vi "Stop Core.vi"(10 "final error code":i32, 11 "ConnectionFactoryHandler in":refnum<class "ConnectionFactoryHandler.lvclass">) -> (3 "ConnectionFactoryHandler out":refnum<class "ConnectionFactoryHandler.lvclass">)   [LabVIEW 2019, in "ConnectionFactorySession.lvlib" / "ConnectionFactoryHandler.lvclass"]
doc: "(<B>Filename</B>: Actor Framework.lvlib:Actor.lvclass:Stop Core.vi)\n\nDefines what the actor does before it stops. Use the <B>final error code</B> input to determine whether the actor shut down in response to an error.\n\nBy default, this method does nothing. A descendant class may override it to define behavior, such as shutting down any processes the actor initiated in its override of the Actor Core method."
uses:
  <vilib>/gpm_packages/@cs/Network-interface/Source/Connection Factory Session/ConnectionFactoryHandler/ConnectionFactoryHandler.lvclass
  <vilib>/gpm_packages/@cs/Network-interface/Source/Connection Factory Session/ConnectionFactoryHandler/ConnectionFactoryHandler.lvclass/ConnectionFactoryHandler.ctl
  <vilib>/gpm_packages/@cs/Network-interface/Source/IConnectionFactory/IConnectionFactory.lvclass
  <vilib>/gpm_packages/@cs/Network-interface/Source/Connection Factory Session/INewConnectionCallback/INewConnectionCallback.lvclass
  <vilib>/gpm_packages/@cs/Network-interface/Source/Logged Actor/LoggedActor.lvclass
  <vilib>/gpm_packages/@cs/Network-interface/Source/Connection Reference/Connection Reference/Connection Reference.lvclass
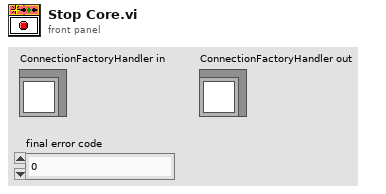
[diagram p1: front panel]
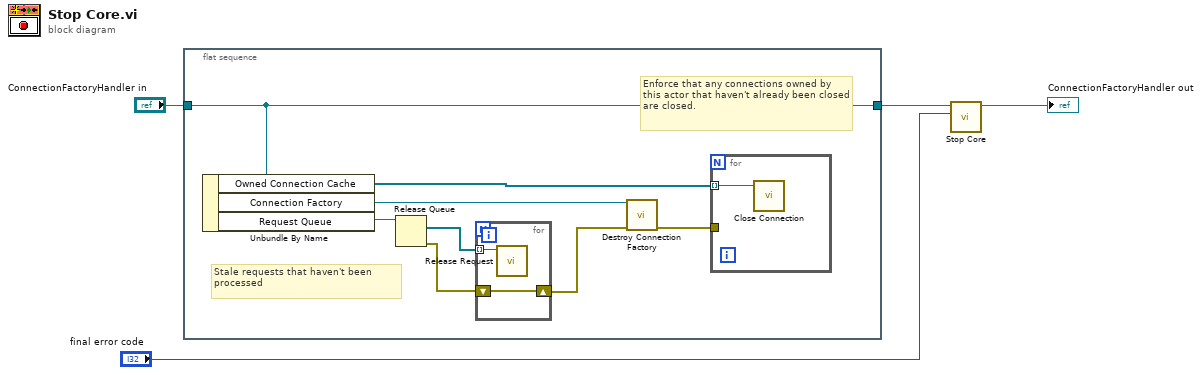
[diagram p0: block diagram]
diagram:
  n1 = flat-sequence {
    tunnel: "ConnectionFactoryHandler in" -> [w10]
    tunnel: [w10] -> w3
    frame #0 {
      # "Enforce that any connections owned by this actor that haven't already been closed are closed."
      # "Stale requests that haven't been processed"
      n2 = Unbundle By Name(w10) -> ("Owned Connection Cache"=w6:refnum<data-value>[], "Connection Factory"=w12:refnum<class "IConnectionFactory.lvclass">, "Request Queue"=w11:refnum<queue>)
      n3 = Release Queue(queue=w11) -> (remaining elements=w9:refnum<class "INewConnectionCallback.lvclass">[], error out=w8:errorcluster)  [unwired: 2 in, 1 out]
      n4 = for {
        tunnel: w9 -> [w15] mode=indexing
        shift-right: [w14] -> w7
        shift-left: w8 -> [w14]
        n5 = call-dynamic "Release Request.vi"("INewConnectionCallback in"=w15) -> ()  [unwired: 11 in]
      }
      n6 = call-dynamic "Destroy Connection Factory.vi"("error in (no error)"=w7, "IConnectionFactory in"=w12) -> ("error out"=w5:errorcluster)  [unwired: 9 in]
      n7 = for {
        tunnel: w6 -> [w13] mode=indexing
        tunnel: w5 -> [_]
        n8 = call <vilib>:"Close Connection.vi"("Connection Reference In"=w13) -> ()  [unwired: 10 in, 1 out]
      }
    }
  }
  n9 = call-parent "Stop Core.vi"("final error code"="final error code", "LoggedActor in"=w3) -> ("LoggedActor out"=→"ConnectionFactoryHandler out":refnum<class "ConnectionFactoryHandler.lvclass">)  [unwired: 9 in]
